vi "CloseAllInstrumentsAtExit.vi"(11 "SpectroscopyUI in":refnum<class "SpectroscopyUI.lvclass">) -> (3 "SpectroscopyUI Out":refnum<class "SpectroscopyUI.lvclass">)   [LabVIEW 2023, in "SpectroscopyUI.lvlib" / "SpectroscopyUI.lvclass"]
uses:
  SpectroscopyUI.lvclass
  SpectroscopyUI.lvclass/SpectroscopyUI.ctl
  <vilib>/ActorFramework/Stop Msg/Stop Msg.lvclass
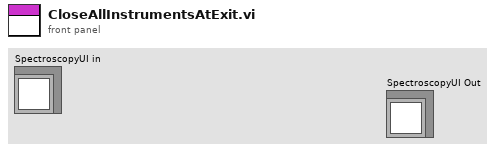
[diagram p1: front panel]
types:
  T1 = typedef "SpectroscopyUI.lvlib/InstrumentData.ctl" = cluster{"Instr Error":errorcluster, "Address":cluster{"address type":enum16{"VISA", "Index"}, "Address":string, "instrument type":T2}, "CurrentState":cluster{"Initialized":bool, "Connected":bool, "Running":bool, "Error":bool}, "Enqueuer":refnum<class "Message Enqueuer.lvclass">}
  T2 = typedef "instrumentType.ctl" = enum16{"Spectrometer", "Camera", "Stepper"}
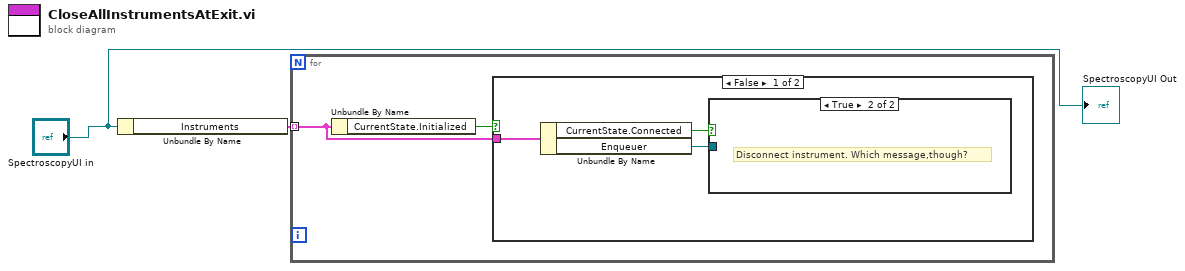
[diagram p0: block diagram]
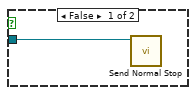
[diagram p2: hidden frame]
diagram:
  n1 = Unbundle By Name("SpectroscopyUI in") -> ("Instruments"=w2:T1[])
  n2 = for {
    tunnel: w2 -> [w3] mode=indexing
    n3 = Unbundle By Name(w3) -> ("CurrentState.Initialized"=w4:bool)
    n4 = case shown="False" w4 {
      tunnel: w3 -> [w7 _]
      frame False {
        n5 = Unbundle By Name(w7) -> ("CurrentState.Connected"=w6:bool, "Enqueuer"=w5:refnum<class "Message Enqueuer.lvclass">)
        n6 = case shown="True" w6 {
          tunnel: w5 -> [w8 _]
          frame False {
            n7 = call <vilib>:"Send Normal Stop.vi"("Message Enqueuer"=w8) -> ()  [unwired: 10 in, 1 out]
          }
          frame True {
            # "Disconnect instrument. Which message,though?"
          }
        }
      }
      frame True {
        # "DeInit instrument. Which message,though?"
      }
    }
  }
  "SpectroscopyUI Out" <- "SpectroscopyUI in"
